vi "Get Config Path.vi"() -> (3 "Config Path":path)   [LabVIEW 2018, in "Config File.lvlib"]
uses:
  Config File.lvlib
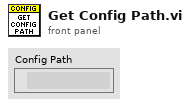
[diagram p1: front panel]
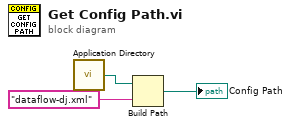
[diagram p0: block diagram]
diagram:
  n1 = call <vilib>:"Application Directory.vi"() -> ("Application Directory"=w3:path)
  n2 = Build Path(base path=w3, name or relative path="dataflow-dj.xml") -> (appended path=→"Config Path":path)
